vi "set_led_enable_test.vi"() -> ()   [LabVIEW 2012]
doc: "This VI is an example of how to use the Host VI to open the I2C bus, write, read, and close I2C bus. This VI should work for any I2C EEPROM or RAM IC. Note that many of these devices have a limit on how many bytes can be writen to the device at a time.\n\nWritten By:\nPeter Fuller\nSenior Engineer\nplf Consulting, LLC\n\nemail: peter@plfconsulting.com\nphone: 617.699.2201"
uses:
  <vilib>/Platform/TimedLoop/XDataNode/timing_clust.ctl
  <vilib>/Platform/TimedLoop/XDataNode/nitl_modes.ctl
  <vilib>/Platform/TimedLoop/XDataNode/wakeup.ctl
  initialization/micron_globals.vi
  <vilib>/Platform/TimedLoop/XDataNode/XDataNode.xnode
  <vilib>/Platform/TimedLoop/XDataNode/XDNodeRunTimeDep.lvlib
panel:
  in  "LED enables":bool[](array[boolean])=[TRUE, TRUE, TRUE, TRUE, TRUE, TRUE]
  in  "Stop":bool
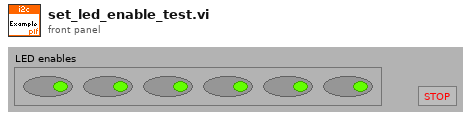
[diagram p1: front panel]
types:
  T1 = typedef "i2c_interface.ctl" = cluster{"FPGA VI Reference":T2}
  T2 = typedef "fpga_reference.ctl" = refnum<k20>
  T3 = typedef "micron_config.ctl" = cluster{"rt fifo":refnum<k33>, "Analog output task":refnum<k21>, "Analog output task 2":refnum<k21>, "Stimulus AO task":refnum<k21>, "Low-rate AIN task":refnum<k21>, "Pedal out task":refnum<k21>, "Pedal in task":refnum<k21>, "Loop timing source":string, "Relay out task":refnum<k21>, "Send UDP Conn":refnum<k16>, "Recv UDP Conn":refnum<k16>, "Host Addr":dbl, "I2C interface":T1, "trace_start notifier":refnum<notifier>, "trace_done notifier":refnum<notifier>, "ASAP FIFO":refnum<k33>}
  T4 = typedef "XDNodeRunTimeDep.lvlib/timing_clust.ctl" = cluster{"Expected End [f-1]":u64, "Actual End [f-1]":u64, "Finished Late? [f-1]":bool, "Expected End [i-1]":u64, "Actual End [i-1]":u64, "Finished Late? [i-1]":bool, "Expected Start [i]":u64, "Actual Start [i]":u64, "Expected Start [f]":u64, "Actual Start [f]":u64, "Source Name":string, "Structure Name":string, "Period":i64, "Deadline":i64, "Offset":i64, "Start":i64, "Priority":i32, "Timeout":i32, "Mode":T5, "Wakeup Reason":T6, "Error":errorcluster, "Source Type":string, "Secondary Source Type":string, "Global End Time":u64, "Global Start Time":u64, "Frame Duration":u64, "Iteration Duration":u64, "Assigned CPU":i32, "I/O Scan Engine Mode":u32}
  T5 = typedef "XDNodeRunTimeDep.lvlib/nitl_modes.ctl" = enum32{"No Change", "Process missed periods, maintain original phase", "Discard missed periods, maintain original phase", "Process missed periods, ignore original phase", "Discard missed periods, ignore original phase"}
  T6 = typedef "XDNodeRunTimeDep.lvlib/wakeup.ctl" = enum32{"Normal", "Aborted", "Asynchronous wakeup", "Timing source error", "Timed loop error", "Timeout"}
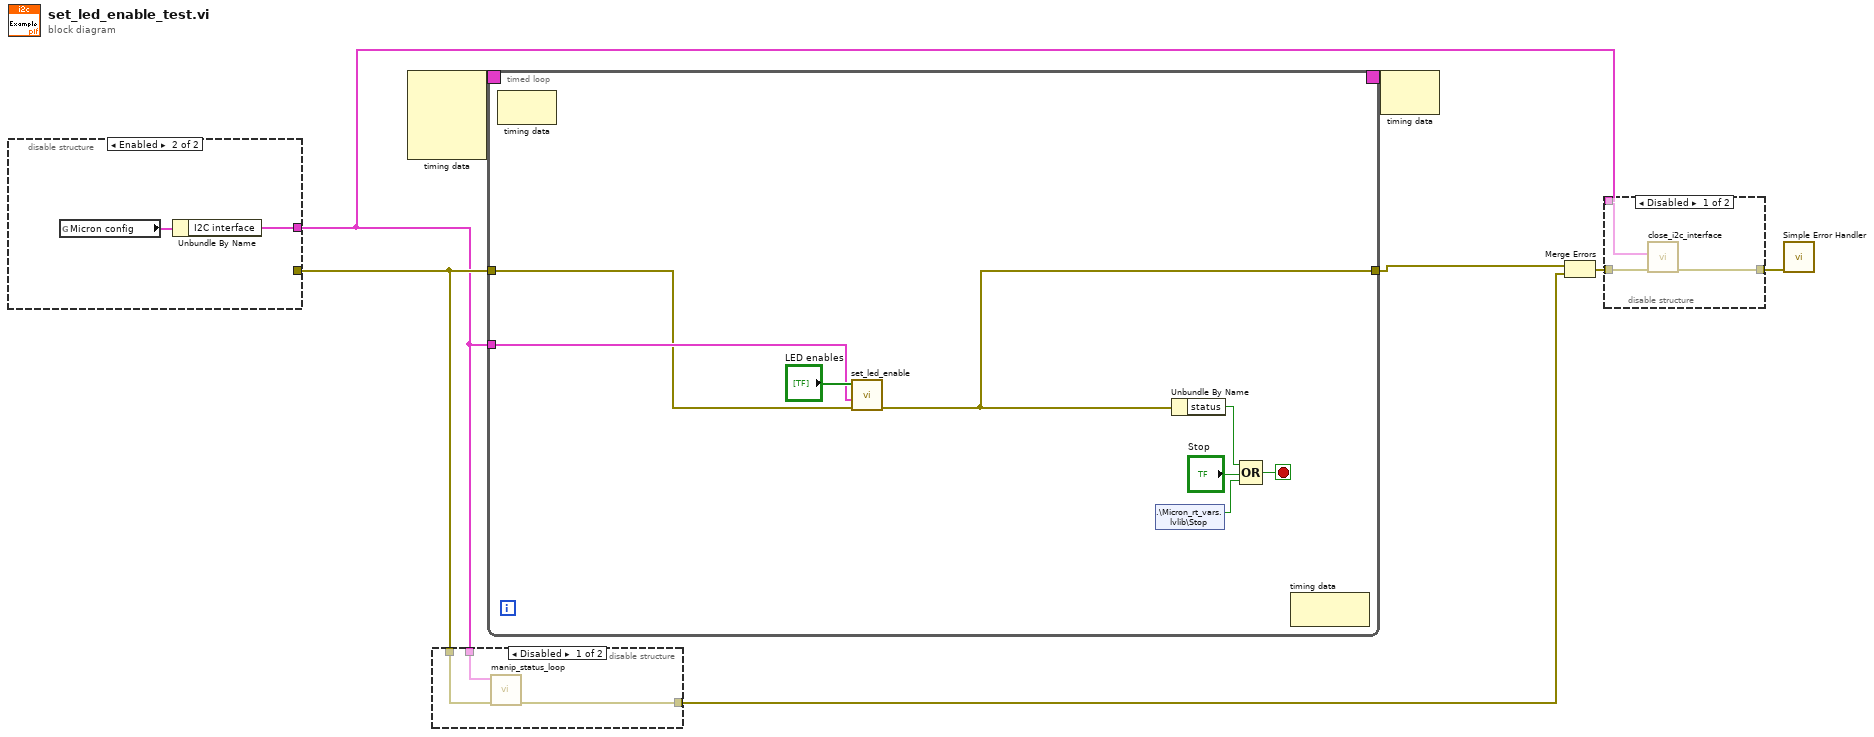
[diagram p0: block diagram]
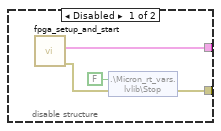
[diagram p3: hidden frame]
diagram:
  n1 = disable-structure shown="Enabled" {
    disable-tunnel: [w10 _] -> w3
    disable-tunnel: [w9 w13] -> w2
    frame Disabled {
      n2 = call "fpga_setup_and_start.vi"() -> ("error out"=w11:errorcluster, "I2C interface"=w9:T1)  [unwired: 10 in]
      n3 = shared-variable ".\\Micron_rt_vars.lvlib\\Stop"(FALSE ("Stop"), error in=w11) -> (error out=w10:errorcluster)
    }
    frame Enabled {
      n4 = global read "micron_globals.vi" "Micron config"() -> (w14:T3)
      n5 = Unbundle By Name(w14) -> ("I2C interface"=w13:T1)
    }
  }
  n6 = node-c288() -> (w7:T4)  [unwired: 4 in]
  n7 = disable-structure shown="Disabled" {
    disable-tunnel: [w17 _] -> w5
    disable-tunnel: w3 -> [w16 _]
    disable-tunnel: w2 -> [w15 _]
    frame Disabled {
      n8 = call "manip_status_loop.vi"("error in"=w16, "I2C interface"=w15) -> ("error out"=w17:errorcluster)  [unwired: 9 in]
    }
    frame Enabled {
    }
  }
  n9 = timed-loop {
    timing: w7 -> [_]
    timing-out: [_] -> w6
    tunnel: w3 -> [w19]
    tunnel: [w18] -> w1
    tunnel: w2 -> [w21]
    stop <- w24 stop-if-true
    n10 = node-c288() -> ()  [unwired: 1 in, 1 out]
    n11 = call "set_led_enable.vi"("error in"=w19, "I2C interface"=w21, "LED enables"="LED enables") -> ("error out"=w18:errorcluster)  [unwired: 8 in]
    n12 = shared-variable ".\\Micron_rt_vars.lvlib\\Stop"() -> (w23:bool)  [unwired: 2 out]
    n13 = Unbundle By Name(w18) -> ("status"=w20:bool)
    n14 = Compound Arithmetic op=OR(w20, "Stop", w23) -> (w24:bool)
    n15 = node-c288() -> ()  [unwired: 1 in, 1 out]
  }
  n16 = node-c288(w6) -> ()  [unwired: 1 out]
  n17 = Merge Errors(w1, w5) -> (w4:errorcluster)
  n18 = disable-structure shown="Disabled" {
    disable-tunnel: [w30 w31] -> w8
    disable-tunnel: w4 -> [w29 w31]
    disable-tunnel: w2 -> [w28 _]
    frame Disabled {
      n19 = call "close_i2c_interface.vi"("error in"=w29, "I2C interface"=w28) -> ("error out"=w30:errorcluster)  [unwired: 9 in]
    }
    frame Enabled {
    }
  }
  n20 = call <vilib>:"Simple Error Handler.vi"("error in (no error)"=w8) -> ()  [unwired: 4 in, 5 out]
